vi "AOTF signals2color.vi"() -> ()   [LabVIEW 2020]
uses:
  <vilib>/DAQmx/write.llb/DAQmx Write (Digital 1D Bool 1Chan 1Samp).vi
  <vilib>/DAQmx/write.llb/DAQmx Write (Analog 1D Wfm NChan NSamp).vi
  <vilib>/DAQmx/create/channels.llb/DAQmx Create Channel (AO-Voltage-Basic).vi
  <vilib>/DAQmx/configure/timing.llb/DAQmx Timing (Use Waveform).vi
  <vilib>/DAQmx/miscellaneous.llb/DAQmx Fill In Error Info.vi
  <vilib>/DAQmx/create/channels.llb/DAQmx Create Channel (DO-Digital Output).vi
  <vilib>/measure/NI_MABase.lvlib
panel:
  out "number of samples written per channel":u32
  in  "Stop":bool
  out "LabVIEW generated Sawtooth input (blue) and Camera trigger (red)":waveform(dbl)[](graph)=[{"t0"=timestamp(0 s since 1904-01-01), "dt"=0.0009854644000985464, "Y"=array[3075 elements]}, {"t0"=timestamp(0 s since 1904-01-01), "dt"=0.0009854644000985464, "Y"=array[3075 elements]}, {"t0"=timestamp(0 s since 1904-01-01), "dt"=0.0009854644000985464, "Y"=array[3075 elements]}]
  out "# Samples written per channel 2":u32=3075
  in  "Stop 2":bool
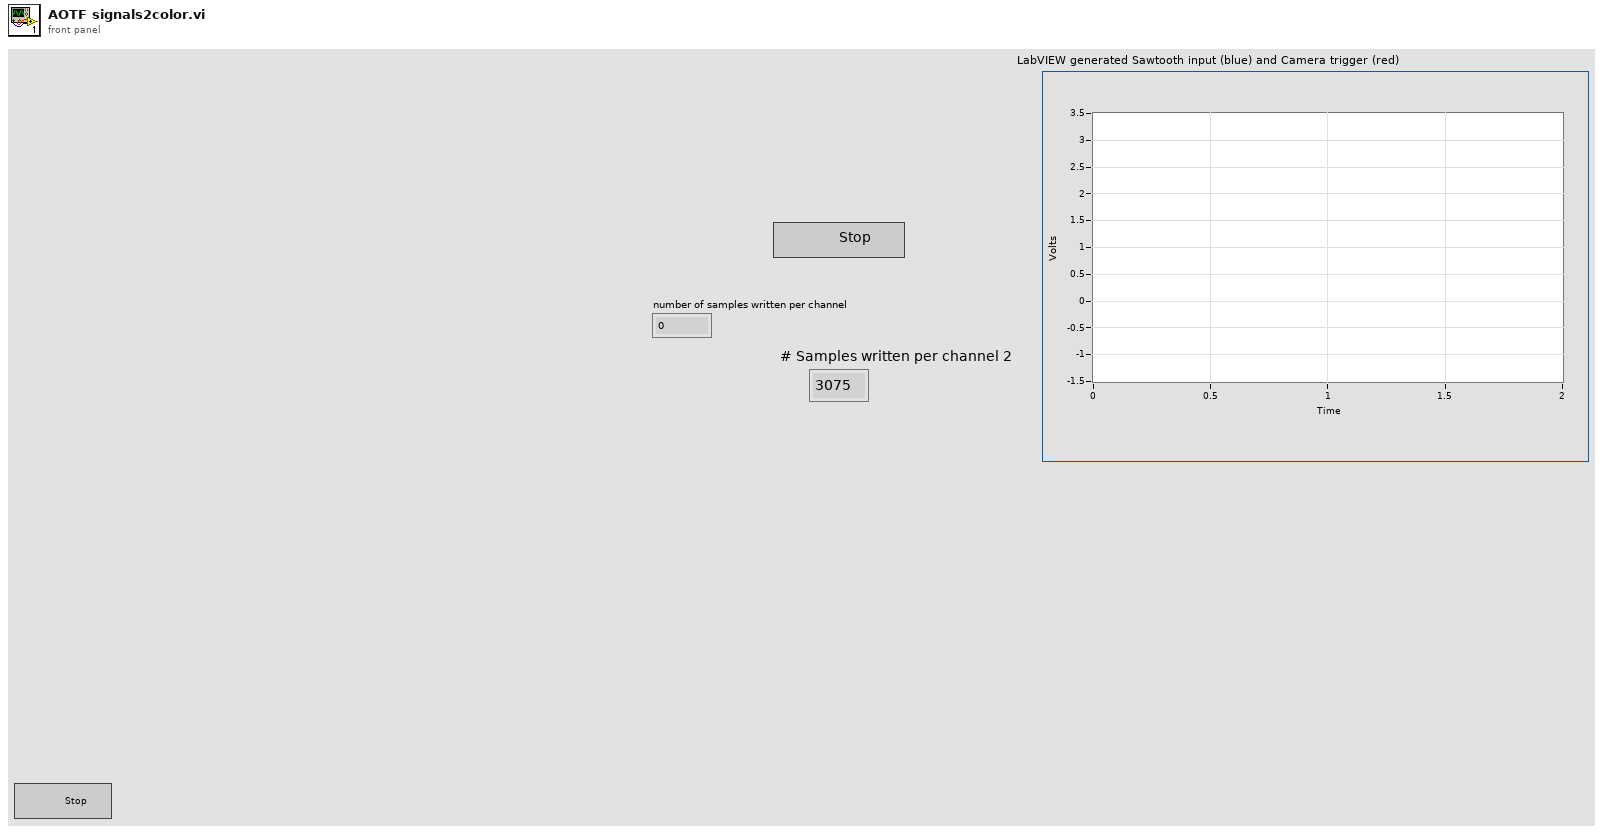
[diagram p1: front panel]
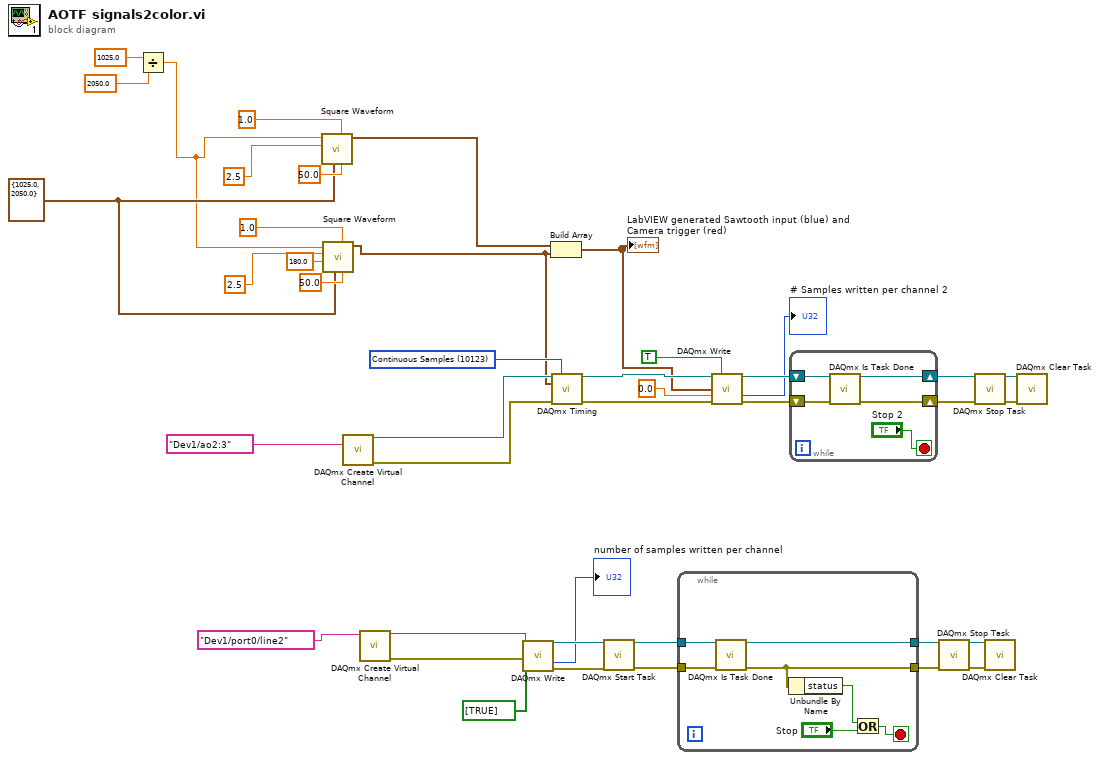
[diagram p0: block diagram]
diagram:
  w15 = cluster{"Fs":dbl, "#s":dbl} {"Fs"=1025.0, "#s"=2050.0} ("sampling info")
  w37 = 10123 items=["Finite Samples"=10178, "Continuous Samples"=10123, "Hardware Timed Single Point"=12522] ("sample mode")
  n1 = Divide(x=1025.0, y=2050.0) -> (x/y=w14:dbl)
  n2 = call <vilib>:"Square Waveform.vi"("duty cycle (%)"=50.0, "offset"=1.0, "sampling info"=w15, "amplitude"=2.5 ("Amplitude for laser 1 (Max value 2.5)"), "frequency"=w14) -> ("signal out"=w23:waveform(dbl))  [unwired: 5 in, 1 out]
  n3 = call <vilib>:"Square Waveform.vi"("duty cycle (%)"=50.0, "offset"=1.0, "sampling info"=w15, "phase"=180.0, "amplitude"=2.5 ("Amplitude for laser 1 (Max value 2.5)"), "frequency"=w14) -> ("signal out"=w19:waveform(dbl))  [unwired: 4 in, 1 out]
  n4 = call-poly <vilib>:"DAQmx Create Virtual Channel.vi"("physical channels"=tag "Dev1/ao2:3") -> ("task out"=w39:refnum<k21>, "error out"=w38:errorcluster)  [unwired: 13 in]
  n5 = call-poly <vilib>:"DAQmx Create Virtual Channel.vi"("lines"=tag "Dev1/port0/line2") -> ("task out"=w13:refnum<k21>, "error out"=w12:errorcluster)  [unwired: 13 in]
  n6 = call-poly <vilib>:"DAQmx Write.vi"("task/channels in"=w13, "data"=bool[] [TRUE], "error in"=w12) -> ("task out"=w11:refnum<k21>, "number of samples written per channel"=→"number of samples written per channel":u32, "error out"=w10:errorcluster)  [unwired: 10 in]
  n7 = Build Array(w23, w19) -> (w27:waveform(dbl)[])
  "LabVIEW generated Sawtooth input (blue) and Camera trigger (red)" <- w27
  n8 = call-poly <vilib>:"DAQmx Timing.vi"("task/channels in"=w39, "sample mode"=w37, "waveform"=w19, "error in"=w38) -> ("task out"=w34:refnum<k21>, "error out"=w33:errorcluster)  [unwired: 10 in]
  n9 = call <vilib>:"DAQmx Start Task.vi"("task/channels in"=w11, "error in"=w10) -> ("task out"=w9:refnum<k21>, "error out"=w8:errorcluster)  [unwired: 12 in]
  n10 = while {
    tunnel: w9 -> [w49]
    tunnel: w8 -> [w48]
    tunnel: [w46] -> w4
    tunnel: [w47] -> w5
    stop <- w43 stop-if-true
    n11 = call <vilib>:"DAQmx Is Task Done.vi"("task/channels in"=w49, "error in"=w48) -> ("task out"=w47:refnum<k21>, "error out"=w46:errorcluster)  [unwired: 11 in, 1 out]
    n12 = Unbundle By Name(w46) -> ("status"=w45:bool)
    n13 = Or(x=w45, y="Stop") -> (x .or. y?=w43:bool)
  }
  n14 = call-poly <vilib>:"DAQmx Write.vi"("task/channels in"=w34, "auto start"=TRUE, "data"=w27, "timeout"=0.0, "error in"=w33) -> ("task out"=w35:refnum<k21>, "number of samples written per channel"=→"# Samples written per channel 2":u32, "error out"=w36:errorcluster)  [unwired: 8 in]
  n15 = while {
    shift-right: [w51] -> w31
    shift-left: w35 -> [w54]
    shift-right: [w52] -> w32
    shift-left: w36 -> [w53]
    stop <- "Stop 2" stop-if-true
    n16 = call <vilib>:"DAQmx Is Task Done.vi"("task/channels in"=w54, "error in"=w53) -> ("task out"=w51:refnum<k21>, "error out"=w52:errorcluster)  [unwired: 11 in, 1 out]
  }
  n17 = call <vilib>:"DAQmx Stop Task.vi"("task/channels in"=w5, "error in"=w4) -> ("task out"=w7:refnum<k21>, "error out"=w6:errorcluster)  [unwired: 12 in]
  n18 = call <vilib>:"DAQmx Stop Task.vi"("task/channels in"=w31, "error in"=w32) -> ("task out"=w40:refnum<k21>, "error out"=w41:errorcluster)  [unwired: 12 in]
  n19 = call <vilib>:"DAQmx Clear Task.vi"("task in"=w7, "error in"=w6) -> ()  [unwired: 13 in, 1 out]
  n20 = call <vilib>:"DAQmx Clear Task.vi"("task in"=w40, "error in"=w41) -> ()  [unwired: 13 in, 1 out]
